vi "Display Warning.vi"(11 "error in (no error)":errorcluster) -> (15 "error out":errorcluster)   [LabVIEW 2015]
uses:
  Exceptions/Exception Warning/Exception Warning.lvclass
  <userlib>/LV Exceptions v1/SubVIs/Catch Single Exception.vi
  <userlib>/LV Exceptions v1/Exception/Exception.lvclass
  <userlib>/LV Exceptions v1/LV Exceptions v1.lvlib
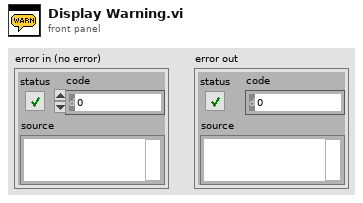
[diagram p1: front panel]
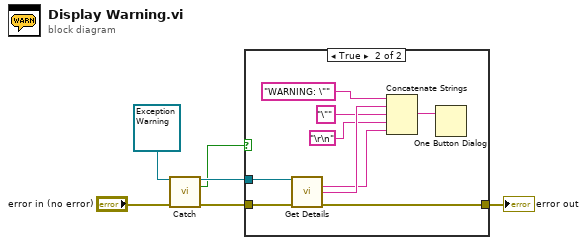
[diagram p0: block diagram]
diagram:
  n1 = call-poly <userlib>:"Catch.vi"("target"=refnum<class "Exception Warning.lvclass"> refnum ("Exception Warning.lvclass"), "error in (no error)"="error in (no error)") -> ("catched exception out"=w4:refnum<class "Exception.lvclass">, "catched"=w1:bool, "error out"=w5:errorcluster)  [unwired: 11 in]
  n2 = case shown="True" w1 {
    tunnel: [w7 w16] -> w6
    tunnel: w5 -> [w7 w15]
    tunnel: w4 -> [_ w14]
    frame False {
    }
    frame True {
      n3 = call-dynamic "Get Details.vi"("exception in"=w14, "error in (no error)"=w15) -> ("message"=w9:string, "class name"=w13:string, "error out"=w16:errorcluster)  [unwired: 8 in, 3 out]
      n4 = Concatenate Strings("WARNING: \"" ("string"), w13, "\"" ("string"), "\r\n", w9) -> (w11:string)
      n5 = One Button Dialog(message=w11) -> ()  [unwired: 1 in, 1 out]
    }
  }
  "error out" <- w6
